vi "Clone Dialog.vi"() -> ()   [LabVIEW 2020, in "MacroAssert Tests.lvlib"]
uses:
  MacroAssert Tests.lvlib
panel:
  out "VI Clone Name":string
  in  "Middle Button":bool
  in  "Right Button":bool
  in  "Left Button":bool
  # "This dialog is a clone"
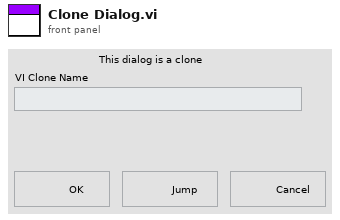
[diagram p1: front panel]
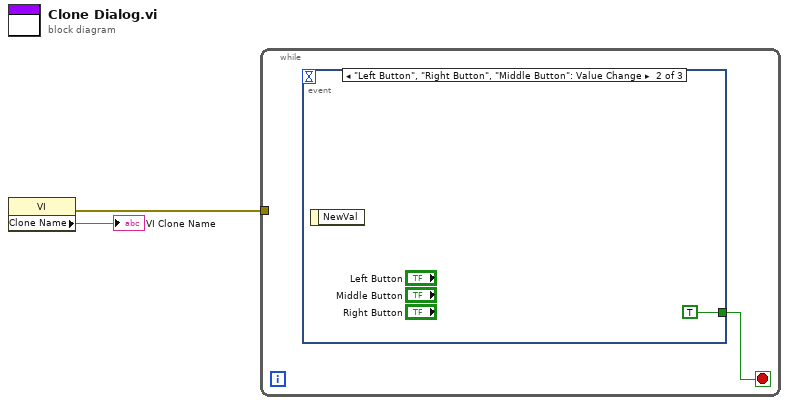
[diagram p0: block diagram]
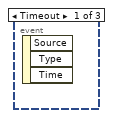
[diagram p2: hidden frame]
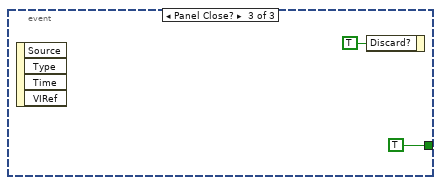
[diagram p3: hidden frame]
diagram:
  n1 = property class="VI"() -> (error out=w1:errorcluster, "Clone Name"=→"VI Clone Name":string)  [unwired: 2 in, 1 out]
  n2 = while {
    tunnel: w1 -> [_]
    stop <- w3 stop-if-true
    n3 = event shown="[1] \"Left Button\", \"Right Button\", \"Middle Button\": Value Change" {
      selector: _ -> [_ _ _]
      dyn-events: _ -> [_ _ _]
      timeout: _ -> [_ _ _]
      tunnel: [_ TRUE TRUE] -> w3
      event Timeout {
        n4 = event-data() -> ()  [unwired: 1 in, 3 out]
      }
      event "Left Button", "Right Button", "Middle Button": Value Change {
        n5 = event-data() -> ()  [unwired: 1 in, 1 out]
      }
      event Panel Close? {
        n6 = event-data() -> ()  [unwired: 1 in, 4 out]
        n7 = event-data("Discard?"=TRUE) -> ()  [unwired: 1 in, 1 out]
      }
    }
  }
